vi "Compute Peak Max Image.vi"(8 "Error In":errorcluster, 9 "Image Array":T1[](array[typedef]), 11 "Image Max in":T1) -> (0 "Error Out":errorcluster, 1 "CPU (s)":dbl, 3 "Image Max out":T1)   [LabVIEW 2021, in "Image.lvlib"]
uses:
  Image.lvlib
  <vilib>/vision/Image Controls.llb/IMAQ Image.ctl
  Image Characteristics.ctl
  Time/Time.lvlib
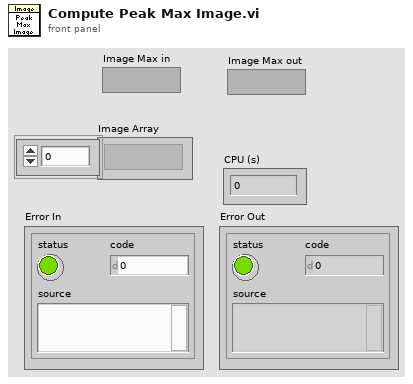
[diagram p1: front panel]
types:
  T1 = typedef "IMAQ Image.ctl" = refnum<image>
  T2 = typedef "Image.lvlib/Image Characteristics.ctl" = cluster{"Calibration":T3, "File Type":string, "X Resolution":i32, "Y Resolution":i32, "File Data Type":i32, "Image Type":T5}
  T3 = typedef "Simple Grid Descriptor" = cluster{"X Step":sgl, "Y Step":sgl, "Unit":T4}
  T4 = typedef "Image Unit" = enum32{"Undefined", "Angström", "Micrometer", "Millimeter", "Centimeter", "Meter", "Kilometer", "Microinch", "Inch", "Feet", "Nautical miles", "Standard miles", "Steps"}
  T5 = typedef "Image Type" = u32
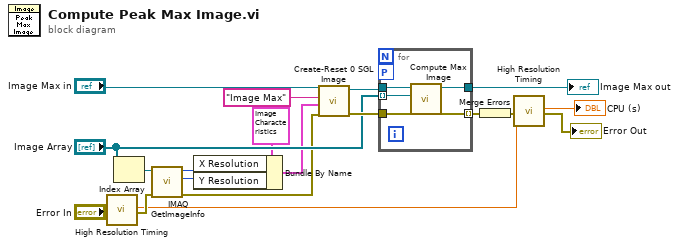
[diagram p0: block diagram]
diagram:
  n1 = call "High Resolution Timing.vi"("Error In"="Error In") -> ("elapsed (relative) seconds"=w4:dbl, "Error Out"=w6:errorcluster)  [unwired: 16 in, 1 out]
  n2 = Index Array(array="Image Array") -> (element=w12:T1)  [unwired: 1 in]
  n3 = call "IMAQ GetImageInfo"("error in (no error)"=w6, "Image"=w12) -> ("error out"=w7:errorcluster, "Y Resolution"=w9:i32, "X Resolution"=w10:i32)  [unwired: 2 in, 5 out]
  n4 = Bundle By Name(cluster=T2 {"Calibration"={"X Step"=0.0, "Y Step"=0.0, "Unit"=enum."Undefined"}, "File Type"="", "X Resolution"=0, "Y Resolution"=0, "File Data Type"=0, "Image Type"=0} ("Image Characteristics"), "X Resolution"=w10, "Y Resolution"=w9) -> (w8:T2)
  n5 = call "Create-Reset 0 SGL Image.vi"("Error In"=w7, "Image Characteristics"=w8, "Image Name"="Image Max", "Image"="Image Max in") -> ("Error Out"=w15:errorcluster, "New Image"=w17:T1)  [unwired: 6 in]
  n6 = for {
    tunnel: "Image Array" -> [w20] mode=indexing
    tunnel: w17 -> [w23]
    tunnel: [w24] -> w19
    tunnel: w15 -> [w22]
    tunnel: [w21] -> w14 mode=indexing
    workers-P: _ -> [_]
    n7 = call "Compute Max Image.vi"("error in (no error)"=w22, "New Image"=w20, "Max Image Dst"=w23) -> ("error out"=w21:errorcluster, "Max Image"=w24:T1)  [unwired: 7 in]
  }
  "Image Max out" <- w19
  n8 = Merge Errors(w14) -> (w1:errorcluster)
  n9 = call "High Resolution Timing.vi"("relative seconds (NaN)"=w4, "Error In"=w1) -> ("elapsed (relative) seconds"=→"CPU (s)":dbl, "Error Out"=→"Error Out":errorcluster)  [unwired: 15 in, 1 out]
